vi "DronePi Global Variables.vi"() -> ()   [LabVIEW 2014]
uses:
  SubVI/Ground Station to Aircraft Coms/SubVI/Hardware Driver/Controls/Coms Driver Interface.ctl
  SubVI/Telemetry/Controls/Telemetry Connection Type.ctl
  <vilib>/httpClient/ClientHandle.ctl
  <vilib>/httpClient/LabVIEWHTTPClient.lvlib
panel:
  out "System Up Time":string
  out "Battery Current":dbl
  out "Status Text":string
  out "Aircraft State":bool
  out "Autotune":bool
  out "Arm":bool
  out "Pos Hold":bool
  out "Stabilise":bool
  out "Altitude Hold":bool
  out "Altitude (m)":dbl
  out "Longitude":dbl
  out "Latitude":dbl
  in  "Aircraft Connection Data":T1
  out "Battery Voltage":dbl
  out "Land":bool
  out "RTL":bool
  out "Loiter":bool
  out "Flight Mode":string
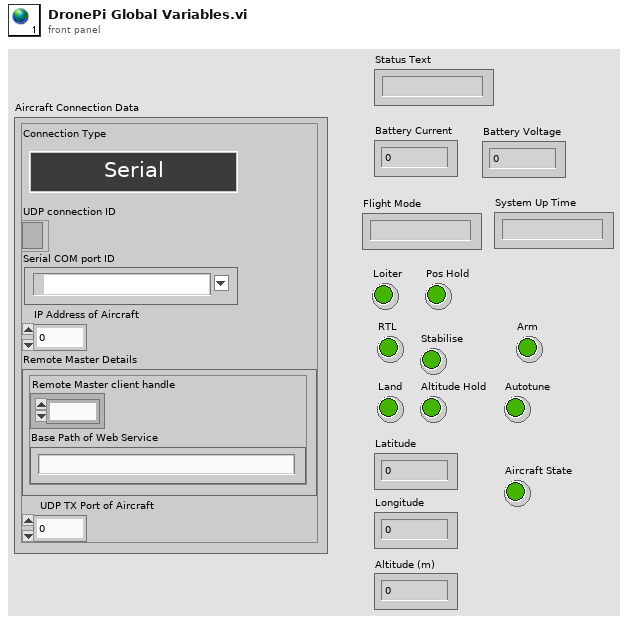
[diagram p1: front panel]
types:
  T1 = typedef "Coms Driver Interface.ctl" = cluster{"Connection Type":T2, "UDP connection ID":refnum<k16>, "Serial COM port ID":refnum<visa-resource-name>, "IP Address of Aircraft":u32, "Remote Master Details":cluster{"Remote Master client handle":T3, "Base Path of Web Service":string}, "UDP TX Port of Aircraft":u16}
  T2 = typedef "Telemetry Connection Type.ctl" = enum16{"Serial", "UDP", "Remote Master"}
  T3 = typedef "LabVIEWHTTPClient.lvlib/ClientHandle.ctl" = refnum<k1>
diagram:
